vi "_API_BINANCE_GET_USDT_FUTURES_minQty.vi"(0 "BinanceAPI in":refnum<class "BinanceAPI_.lvclass">, 5 "minQantity":cluster{"symbol (eg. BTCUSDT)":string}={"symbol (eg. BTCUSDT)"="XRPUSDT"}, 11 "error in (no error)":errorcluster) -> (4 "BinanceAPI out":refnum<class "BinanceAPI_.lvclass">, 6 "min Quantity":dbl format="%#.6f", 15 "error out":errorcluster)   [LabVIEW 2022 SP3, in "BinanceAPI_.lvclass"]
doc: "https://binance-docs.github.io/apidocs/futures/en/#exchange-information\n\n\nOnly <B>minimal quantity</B> (minqty)"
uses:
  BinanceAPI_.lvclass
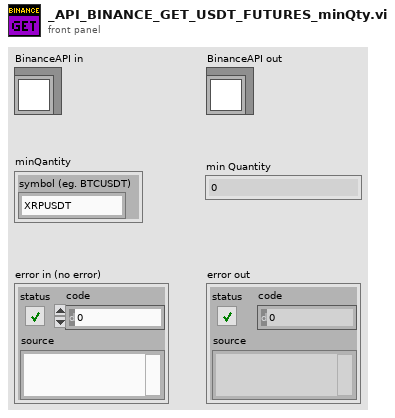
[diagram p1: front panel]
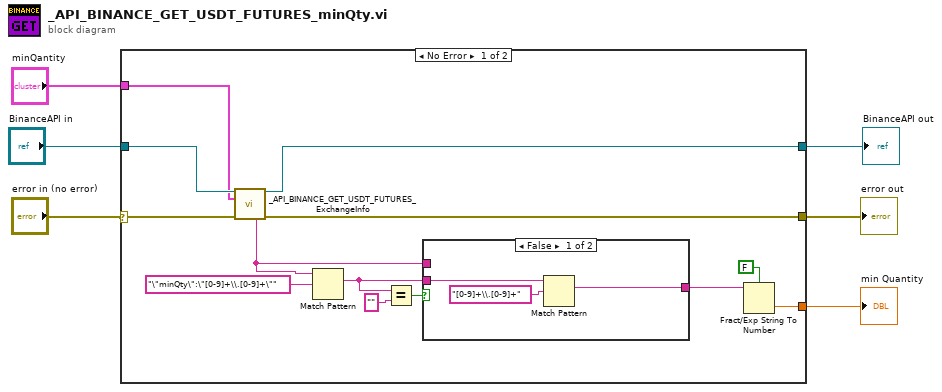
[diagram p0: block diagram]
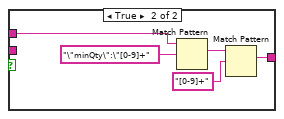
[diagram p2: hidden frame]
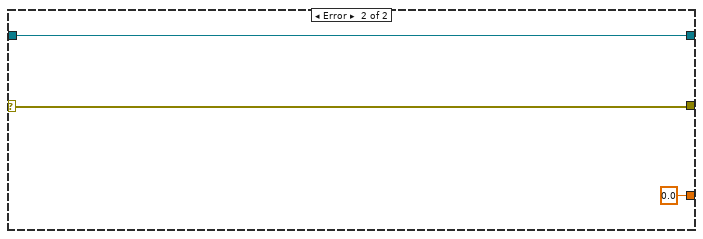
[diagram p3: hidden frame]
diagram:
  n1 = case shown="No Error" "error in (no error)" {
    selector: "error in (no error)" -> [w8 w29]
    tunnel: [w18 w29] -> w6
    tunnel: "BinanceAPI in" -> [w17 w30]
    tunnel: [w16 w30] -> w1
    tunnel: [w12 0.0] -> w5
    tunnel: "minQantity" -> [w7 _]
    frame No Error {
      n2 = call "_API_BINANCE_GET_USDT_FUTURES_ExchangeInfo.vi"("BinanceAPI in"=w17, "exchangeInfo"=w7, "error in (no error)"=w8) -> ("BinanceAPI out"=w16:refnum<class "BinanceAPI_.lvclass">, "insideInfo"=w19:string, "error out"=w18:errorcluster)  [unwired: 8 in, 2 out]
      n3 = Match Pattern(string=w19, regular expression="\"minQty\":\"[0-9]+\\.[0-9]+\"") -> (match substring=w10:string)  [unwired: 1 in, 3 out]
      n4 = Equal?(x=w10, y="" ("match substring")) -> (x = y?=w9:bool)
      n5 = case shown="False" w9 {
        tunnel: [w21 w24] -> w14
        tunnel: w10 -> [w20 _]
        tunnel: w19 -> [_ w23]
        frame False {
          n6 = Match Pattern(string=w20, regular expression="[0-9]+\\.[0-9]+") -> (match substring=w21:string)  [unwired: 1 in, 3 out]
        }
        frame True {
          n7 = Match Pattern(string=w23, regular expression="\"minQty\":\"[0-9]+") -> (match substring=w25:string)  [unwired: 1 in, 3 out]
          n8 = Match Pattern(string=w25, regular expression="[0-9]+") -> (match substring=w24:string)  [unwired: 1 in, 3 out]
        }
      }
      n9 = Fract/Exp String To Number(use system decimal point (T)=FALSE, string=w14) -> (number=w12:dbl)  [unwired: 2 in, 1 out]
    }
    frame Error {
    }
  }
  "min Quantity" <- w5
  "error out" <- w6
  "BinanceAPI out" <- w1
